vi "FTW-CodeGen-GenerateCode.vi"(0 "State In":T2, 5 "XRef":refnum<vi>, 7 "Terms":T1(array[cluster]), 9 "Diagram":refnum<vi>) -> (4 "State Out":T2, 6 "Reply":string[](array[string]), 8 "Generated Code?":bool)   [LabVIEW 2015, in "FTW-dotNet-SQL-Insert.xnode"]
uses:
  FTW-dotNet-SQL-Insert.xnode
  FTW-CodeGen-State.ctl
  src/reflection/FTW-Reflection-Type.vi
  src/regex/FTW-Regex-Execute.vi
  src/error/FTW-ERR-ThrowError.vi
  src/error/FTW-ERR-ThrowGenericError.vi
  src/error/FTW-ERR-CallChain.vi
  src/error/FTW-ERR-NoErrorConstant.vi
  src/string/FTW-STR-ReplaceWhitespace.vi
  src/string/FTW-STR-Array-Delimit.vi
  src/error/FTW-ERR-Clear.vi
  src/regex/FTW-Regex-ReplaceAll.vi
  src/regex/FTW-Regex-Construct.vi
  lib/FTW-KernelFilepath.vi
  src/regex/FTW-Regex-Destroy.vi
panel:
  # "Inputs"
  # "Outputs"
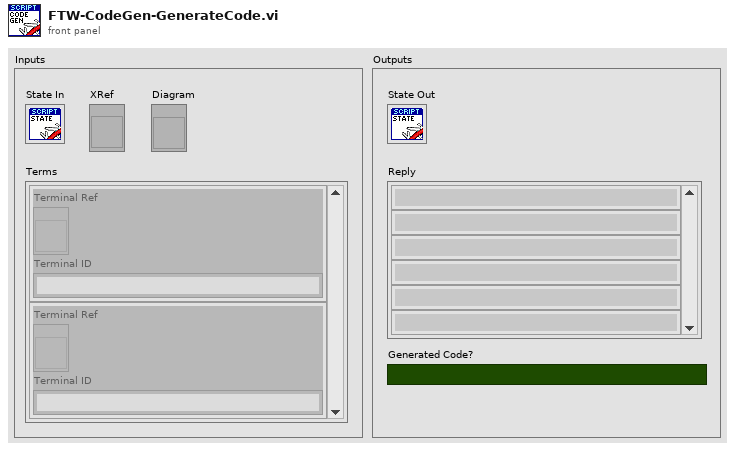
[diagram p1: front panel]
types:
  T1 = cluster{"Terminal Ref":refnum<vi>, "Terminal ID":string}[]
  T2 = typedef "FTW-dotNet-SQL-Insert.xnode/FTW-CodeGen-State.ctl" = cluster{"Dummy":string}
  T3 = typedef "LVPositionTypeDef.ctl" = cluster{"Left":i32, "Top":i32}
  T4 = typedef "FTW-Reflection-Types.ctl" = enum16{"Unknown", "Void", "Array", "Cluster", "LVObject", "Boolean", "I8", "I16", "I32", "I64", "U8", "U16", "U32", "U64", "SGL", "DBL", "EXT", "CSG", "CDB", "CXT", "FXP", "EnumU8", "EnumU16", "EnumU32", "EnumU64", "SGLwithUnit", "DBLwithUnit", "EXTwithUnit", "CSGwithUnit", "CDBwithUnit", "CXTwithUnit", "String", "Path", "Picture", "Tag", "LVVariant", "Timestamp", "WaveformI8", "WaveformI16", "WaveformI32", "WaveformI64", "WaveformU8", "WaveformU16", "WaveformU32", "WaveformU64", "WaveformSGL", "WaveformDBL", "WaveformEXT", "WaveformCSG", "WaveformCDB", "WaveformCXT", "WaveformDigital", "WaveformUnknownType", "DigitalData", "DynamicData", "ExternalData", "FileByteStream", "TDMStream", "dotNET", "ActiveX", "VIServerReference", "VIReference", "ApplicationInstance", "Menu", "ConnectionDataSocket", "ConnectionVISA", "ConnectionBluetooth", "ConnectionIrDA", "ConnectionTCP", "ConnectionUDP", "ConnectionHTTPClient", "ConnectionFTP", "Occurrence", "Notifier", "Queue", "Rendezvous", "Semaphore", "RTFIFO", "EventPublisher", "EventRegistration", "EventCallback", "DataValueReference", "GenericClass", "GenericClassTag", "GenericClassDeepCopy", "GenericClassFlattened", "GenericClassTagFlattened", "GenericReferenceType", "WindowsRegistry", "OverloadedDatalogRef", "ReferenceUnknownType", "ByteArray", "ConPaneInterface"}
  T5 = cluster{"Element Name":string, "Element Type":T4, "Element Value":variant}[]
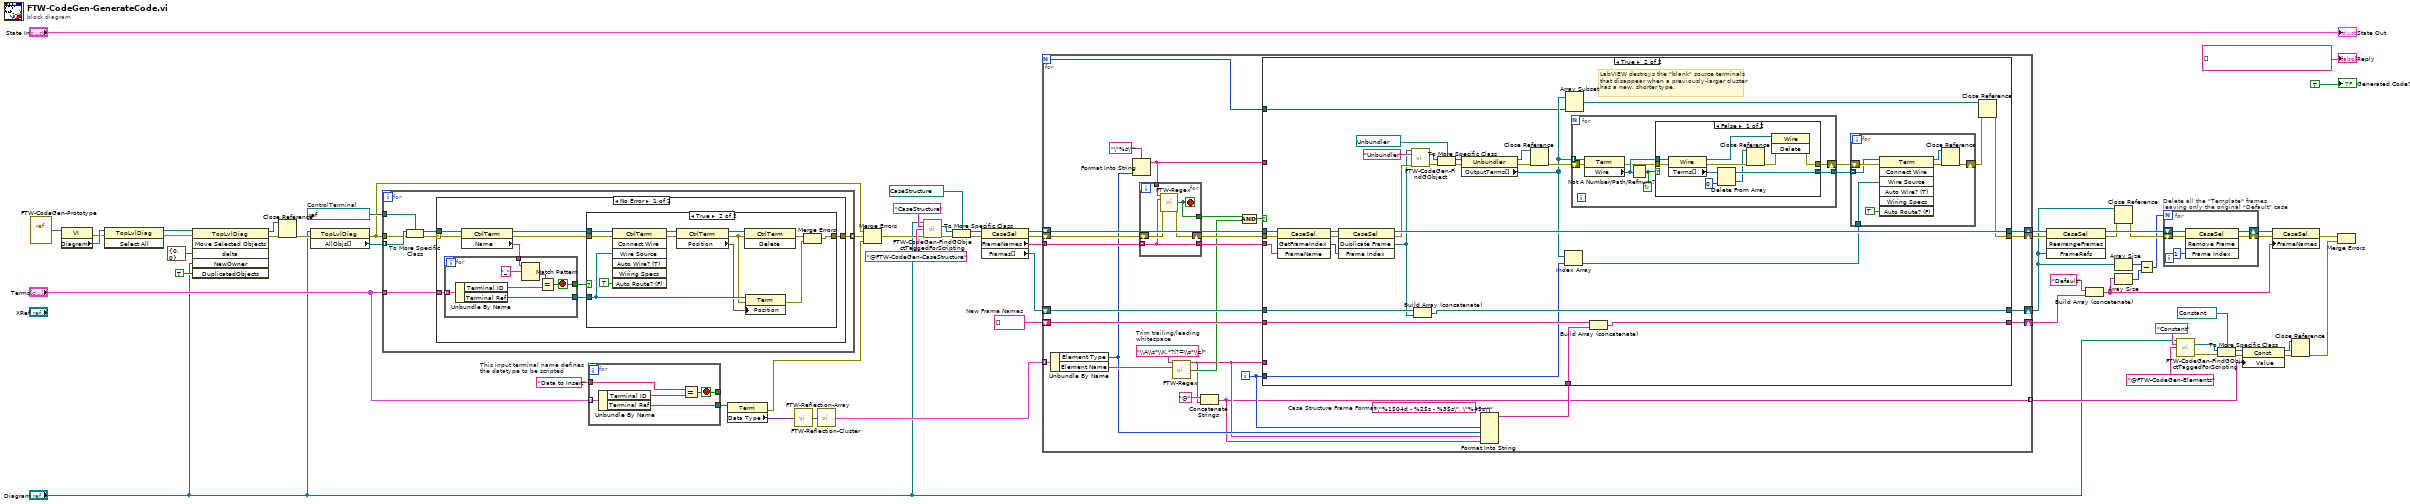
[diagram p0: block diagram]
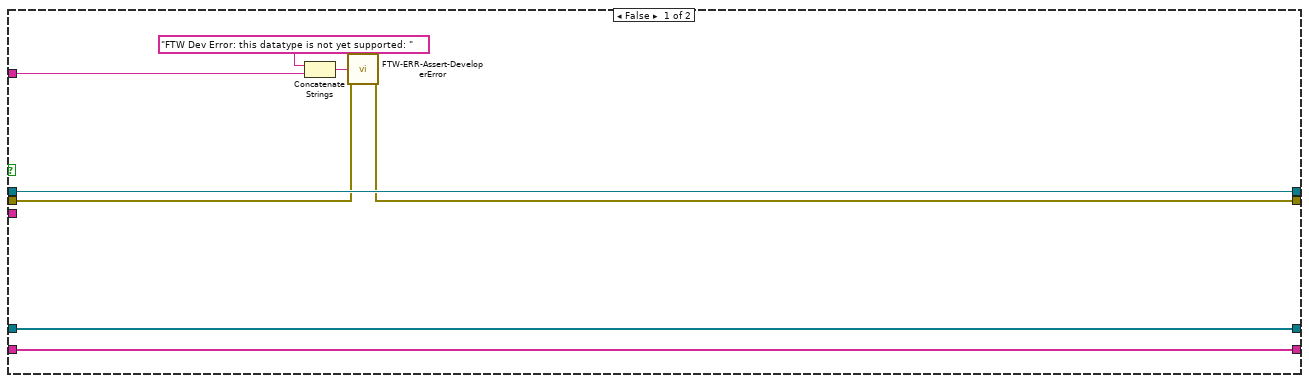
[diagram p2: hidden frame]
diagram:
  w30 = string[] []  # New Frame Names
  w42 = "Data to Insert"  # This input terminal name defines the datatype to be scripted
  w59 = refnum<vi> refnum  # ControlTerminal
  n1 = vi-ref "FTW-CodeGen-Prototype.vi"() -> (w52:refnum<vi>)
  n2 = property class="VI"(reference=w52) -> (error out=w51:errorcluster, "Diagram"=w58:refnum<vi>)  [unwired: 1 in, 1 out]
  n3 = invoke class="TopLvlDiag" method="Select All"(reference=w58, error in=w51) -> (reference out=w62:refnum<vi>, error out=w61:errorcluster)  [unwired: 1 in, 1 out]
  n4 = invoke class="TopLvlDiag" method="Move Selected Objects"(reference=w62, error in=w61, "delta"=cluster{"X":i32, "Y":i32} {"X"=0, "Y"=0} ("X/Y Delta"), "NewOwner"="Diagram", "DuplicatedObjects"=TRUE ("Duplicate? (F)")) -> (reference out=w48:refnum<vi>, error out=w50:errorcluster)  [unwired: 1 in, 4 out]
  n5 = Close Reference(reference=w48, error in (no error)=w50) -> (error out=w49:errorcluster)
  n6 = property class="TopLvlDiag"(reference="Diagram", error in=w49) -> (error out=w56:errorcluster, "AllObjs[]"=w60:refnum<vi>[])  [unwired: 1 out]
  n7 = for {
    tunnel: w60 -> [w71] mode=indexing
    tunnel: w56 -> [w70]
    tunnel: w59 -> [w69]
    tunnel: "Terms" -> [w66]
    tunnel: [w65] -> w57 mode=indexing
    n8 = To More Specific Class(target class=w69, reference=w71, error in=w70) -> (specific class reference=w67:refnum<vi>, error out=w68:errorcluster)
    n9 = case shown="No Error" w68 {
      selector: w68 -> [w79 _]
      tunnel: w67 -> [w80 _]
      tunnel: w66 -> [w78 _]
      tunnel: [w73 _] -> w65
      frame No Error {
        n10 = property class="CtrlTerm"(reference=w80, error in=w79) -> (reference out=w75:refnum<vi>, error out=w74:errorcluster, "Name"=w77:string)
        n11 = for {
          tunnel: w78 -> [w100] mode=indexing
          tunnel: w77 -> [w98]
          tunnel: [w99] -> w76
          tunnel: [w94] -> w72
          stop <- w94 stop-if-true
          n12 = Unbundle By Name(w100) -> ("Terminal ID"=w95:string, "Terminal Ref"=w99:refnum<vi>)
          n13 = Match Pattern(string=w98, regular expression="_") -> (after substring=w96:string)  [unwired: 1 in, 3 out]
          n14 = Equal?(x=w96, y=w95) -> (x = y?=w94:bool)
        }
        n15 = case shown="True" w72 {
          tunnel: w76 -> [_ w85]
          tunnel: w75 -> [_ w93]
          tunnel: w74 -> [w81 w92]
          tunnel: [w81 w87] -> w73
          frame False {
          }
          frame True {
            n16 = invoke class="CtrlTerm" method="Connect Wire"(reference=w93, error in=w92, "Wire Source"=w85, "Auto Route? (F)"=TRUE) -> (reference out=w91:refnum<vi>, error out=w89:errorcluster)  [unwired: 3 in, 5 out]
            n17 = property class="CtrlTerm"(reference=w91, error in=w89) -> (reference out=w90:refnum<vi>, error out=w84:errorcluster, "Position"=w82:T3)
            n18 = invoke class="CtrlTerm" method="Delete"(reference=w90, error in=w84) -> (error out=w88:errorcluster)  [unwired: 1 in, 2 out]
            n19 = property class="Term"(reference=w85, error in=w84, "Position"=w82) -> (error out=w83:errorcluster)  [unwired: 1 out]
            n20 = Merge Errors(w88, w83) -> (w87:errorcluster)
          }
        }
      }
      frame Error {
      }
    }
  }
  n21 = for {
    tunnel: "Terms" -> [w105] mode=indexing
    tunnel: [w104] -> w40
    tunnel: [w102] -> _
    tunnel: w42 -> [w101]
    stop <- w102 stop-if-true
    n22 = Unbundle By Name(w105) -> ("Terminal ID"=w103:string, "Terminal Ref"=w104:refnum<vi>)
    n23 = Equal?(x=w101, y=w103) -> (x = y?=w102:bool)
  }
  n24 = property class="Term"(reference=w40) -> (error out=w15:errorcluster, "Data Type"=w14:variant)  [unwired: 1 in, 1 out]
  n25 = call "FTW-Reflection-Array.vi"("Array"=w14) -> ("Default Array Element"=w13:variant)  [unwired: 13 in, 1 out]
  n26 = call "FTW-Reflection-Cluster.vi"("Cluster"=w13) -> ("Cluster Elements"=w39:T5)  [unwired: 14 in]
  n27 = Merge Errors(w56, w57, w15) -> (w46:errorcluster)
  n28 = call "FTW-CodeGen-FindGObjectTaggedForScripting.vi"("GObject to Traverse"="Diagram", "Class Name"="CaseStructure", "Label Prefix to uniquely identify node"="@FTW-CodeGen-CaseStructure" ("Label to uniquely identify node"), "error in"=w46) -> ("GObject"=w45:refnum<vi>, "error out"=w44:errorcluster)  [unwired: 9 in, 1 out]
  n29 = To More Specific Class(target class=refnum<vi> refnum ("Object"), reference=w45, error in=w44) -> (specific class reference=w38:refnum<vi>, error out=w36:errorcluster)
  n30 = property class="CaseSel"(reference=w38, error in=w36) -> (reference out=w37:refnum<vi>, error out=w35:errorcluster, "FrameNames"=w34:string[], "Frames[]"=w22:refnum<vi>[])
  n31 = for {
    N -> [w114]
    tunnel: w39 -> [w130] mode=indexing
    tunnel: w34 -> [w120]
    shift-right: [w125] -> w27
    shift-left: w37 -> [w132]
    shift-right: [w126] -> w25
    shift-left: w35 -> [w131]
    shift-right: [w124] -> w21
    shift-left: w22 -> [w127]
    shift-right: [w122] -> w28
    shift-left: w30 -> [w123]
    tunnel: [w107] -> w3 mode=indexing
    i -> [w112]
    w106 = "\"%1$04d - %2$s - %3$s\", \"%4$s\""  # Case Structure Frame Format
    w118 = "\\A\\s*\\K.*?(?=\\s*\\z)"  # Trim trailing/leading whitespace
    n32 = Unbundle By Name(w130) -> ("Element Type"=w110:T4, "Element Name"=w113:string)
    n33 = Format Into String(format string="\"%s\"", w110) -> (resulting string=w128:string)  [unwired: 2 in, 1 out]
    n34 = for {
      tunnel: w128 -> [w136]
      shift-right: [w135] -> w121
      shift-left: w131 -> [w137]
      tunnel: w120 -> [w133] mode=indexing
      tunnel: [w134] -> w117
      tunnel: [w133] -> w119
      stop <- w134 stop-if-true
      n35 = call "FTW-Regex.vi"("Regular Expression"=w136, "Input String"=w133, "error in"=w137) -> ("Match Found?"=w134:bool, "error out"=w135:errorcluster)  [unwired: 8 in, 3 out]
    }
    n36 = call "FTW-Regex.vi"("Regular Expression"=w118, "Input String"=w113) -> ("Match"=w108:string, "Match Found?"=w115:bool)  [unwired: 9 in, 3 out]
    n37 = Concatenate Strings("@" ("string"), w108) -> (w107:string)
    n38 = Compound Arithmetic op=AND(w117, w115) -> (w116:bool)
    n39 = Format Into String(format string=w106, w112, w110, w108, w107) -> (resulting string=w111:string)  [unwired: 2 in, 1 out]
    n40 = case shown="True" w116 {
      tunnel: w121 -> [w139 w172]
      tunnel: w132 -> [w145 w173]
      tunnel: w127 -> [w144 w177]
      tunnel: [w144 w174] -> w124
      tunnel: [w138 w152] -> w126
      tunnel: [w145 w167] -> w125
      tunnel: w123 -> [w143 w176]
      tunnel: [w143 w175] -> w122
      tunnel: w119 -> [_ w168]
      tunnel: w108 -> [_ _]
      tunnel: w112 -> [_ w147]
      tunnel: w128 -> [w141 _]
      tunnel: w114 -> [_ w149]
      tunnel: w111 -> [_ w146]
      frame False {
        n41 = Concatenate Strings("FTW Dev Error: this datatype is not yet supported: " ("Reason this error should never happen"), w141) -> (w140:string)
        n42 = call "FTW-ERR-Assert-DeveloperError.vi"("Reason this error should never happen"=w140, "error in"=w139) -> ("error out"=w138:errorcluster)  [unwired: 13 in]
      }
      frame True {
        # "LabVIEW destroys the \"blank\" source terminals\nthat disappear when a previously-larger cluster\nhas a new, shorter type."
        n43 = invoke class="CaseSel" method="GetFrameIndex"(reference=w173, error in=w172, "FrameName"=w168) -> (reference out=w171:refnum<vi>, error out=w170:errorcluster, "GetFrameIndex"=w169:i32)  [unwired: 1 in, 1 out]
        n44 = invoke class="CaseSel" method="Duplicate Frame"(reference=w171, error in=w170, "Frame Index"=w169) -> (reference out=w167:refnum<vi>, error out=w154:errorcluster, "Duplicate Frame"=w153:refnum<vi>)  [unwired: 1 in, 1 out]
        n45 = call "FTW-CodeGen-FindGObject.vi"("GObject to Traverse"=w153, "Class Name"="Unbundler", "error in"=w154) -> ("GObject"=w164:refnum<vi>, "error out"=w165:errorcluster)  [unwired: 11 in]
        n46 = Build Array (concatenate)(w177, w153) -> (w174:refnum<vi>[])
        n47 = To More Specific Class(target class=refnum<vi> refnum ("Object"), reference=w164, error in=w165) -> (specific class reference=w162:refnum<vi>, error out=w161:errorcluster)
        n48 = property class="Unbundler"(reference=w162, error in=w161) -> (reference out=w156:refnum<vi>, error out=w158:errorcluster, "OutputTerms[]"=w150:refnum<vi>[])
        n49 = Close Reference(reference=w156, error in (no error)=w158) -> (error out=w157:errorcluster)
        n50 = Index Array(array=w150, index=w147) -> (element=w160:refnum<vi>)
        n51 = Array Subset(array=w150, length=w149) -> (w148:refnum<vi>[])  [unwired: 1 in]
        n52 = for {
          tunnel: w150 -> [w191] mode=indexing
          tunnel: [w188] -> w151
          shift-right: [w185] -> w159
          shift-left: w157 -> [w186]
          stop <- w189 continue-if-true
          n53 = property class="Term"(reference=w191, error in=w186) -> (error out=w187:errorcluster, "Wire"=w190:refnum<vi>)  [unwired: 1 out]
          n54 = Not A Number/Path/Refnum?(number/path/refnum=w190) -> (NaN/Path/Refnum?=w189:bool)
          n55 = case shown="False" w189 {
            tunnel: w190 -> [w201 _]
            tunnel: [w199 _] -> w188
            tunnel: w187 -> [w198 w202]
            tunnel: [w196 w202] -> w185
            frame False {
              n56 = property class="Wire"(reference=w201, error in=w198) -> (reference out=w197:refnum<vi>, error out=w195:errorcluster, "Terms[]"=w200:refnum<vi>[])
              n57 = Delete From Array(array=w200, index=0) -> (deleted portion=w193:refnum<vi>, array with subset deleted=w199:refnum<vi>[])  [unwired: 1 in]
              n58 = Close Reference(reference=w193, error in (no error)=w195) -> (error out=w194:errorcluster)
              n59 = invoke class="Wire" method="Delete"(reference=w197, error in=w194) -> (error out=w196:errorcluster)  [unwired: 1 in, 2 out]
            }
            frame True {
            }
          }
        }
        n60 = Build Array (concatenate)(w176, w146) -> (w175:string[])
        n61 = for {
          tunnel: w160 -> [w184]
          shift-right: [w178] -> w155
          shift-left: w159 -> [w182]
          tunnel: w151 -> [w181] mode=indexing
          n62 = invoke class="Term" method="Connect Wire"(reference=w181, error in=w182, "Wire Source"=w184, "Auto Route? (F)"=TRUE) -> (reference out=w180:refnum<vi>, error out=w179:errorcluster)  [unwired: 3 in, 5 out]
          n63 = Close Reference(reference=w180, error in (no error)=w179) -> (error out=w178:errorcluster)
        }
        n64 = Close Reference(reference=w148, error in (no error)=w155) -> (error out=w152:errorcluster)
      }
    }
  }
  n65 = invoke class="CaseSel" method="RearrangeFrames"(reference=w27, error in=w25, "FrameRefs"=w21) -> (reference out=w26:refnum<vi>, error out=w24:errorcluster)  [unwired: 1 in, 2 out]
  n66 = Build Array (concatenate)("Default", w28) -> (w20:string[])
  n67 = Close Reference(reference=w21, error in (no error)=w24) -> (error out=w23:errorcluster)
  n68 = Array Size(array=w21) -> (size(s)=w19:i32)
  n69 = Array Size(array=w20) -> (size(s)=w18:i32)
  n70 = Subtract(x=w19, y=w18) -> (x-y=w17:i32)
  n71 = for "Delete all the \"Template\" frames,\nleaving only the original \"Default\" case" {
    N: w17 -> [_]
    shift-right: [w204] -> w32
    shift-left: w23 -> [w205]
    shift-right: [w206] -> w33
    shift-left: w26 -> [w207]
    n72 = invoke class="CaseSel" method="Remove Frame"(reference=w207, error in=w205, "Frame Index"=u32 1) -> (reference out=w206:refnum<vi>, error out=w204:errorcluster)  [unwired: 1 in, 2 out]
  }
  n73 = call "FTW-CodeGen-FindGObjectTaggedForScripting.vi"("GObject to Traverse"="Diagram", "Class Name"="Constant", "Label Prefix to uniquely identify node"="@FTW-CodeGen-Elements" ("Label to uniquely identify node")) -> ("GObject"=w10:refnum<vi>, "error out"=w9:errorcluster)  [unwired: 10 in, 1 out]
  n74 = To More Specific Class(target class=refnum<vi> refnum ("Object"), reference=w10, error in=w9) -> (specific class reference=w8:refnum<vi>, error out=w7:errorcluster)
  n75 = property class="Const"(reference=w8, error in=w7, "Value"=w3) -> (reference out=w5:refnum<vi>, error out=w4:errorcluster)
  n76 = property class="CaseSel"(reference=w33, error in=w32, "FrameNames"=w20) -> (error out=w16:errorcluster)  [unwired: 1 out]
  n77 = Close Reference(reference=w5, error in (no error)=w4) -> (error out=w1:errorcluster)
  n78 = Merge Errors(w16, w1) -> ()  [unwired: 1 out]
  "State Out" <- "State In"
  "Reply" <- string[] [] ("Reply")
  "Generated Code?" <- TRUE ("Generated Code?")
